vi "URL Read 3.vi"(4 "error in (no error)":errorcluster, 6 "Container State":T3, 7 "Display State In":T1={"WebView2 Ref"=refnum, "event callback refnum"=refnum, "Events"={"Navigation Complete Event"=refnum, "Source Changed Event"=refnum, "Document Title Changed Event"=refnum, "Status Bar Text Changed"=refnum, "Web Message Received"=refnum, "Window Close Requested"=refnum}, "Paths"={"Webview2 Native"=path "C:/Users/kleins/Desktop/webview2/microsoft.web.webview2.1.0.1370.28/build/native", "Edge Application"=path "", "User Data"=path ""}}) -> (0 "error out":errorcluster, 2 "Value":string, 3 "Display State Out":T1={"WebView2 Ref"=refnum, "event callback refnum"=refnum, "Events"={"Navigation Complete Event"=refnum, "Source Changed Event"=refnum, "Document Title Changed Event"=refnum, "Status Bar Text Changed"=refnum, "Web Message Received"=refnum, "Window Close Requested"=refnum}, "Paths"={"Webview2 Native"=path "C:/Users/kleins/Desktop/webview2/microsoft.web.webview2.1.0.1370.28/build/native", "Edge Application"=path "", "User Data"=path ""}})   [LabVIEW 2020, in "WebView2 Control.xctl"]
uses:
  WebView2 Control.xctl
  <vilib>/_xctls/Container State.ctl
  State.ctl
  E:/Labview/LV 2020/Libs/LV-WebView2/microsoft.web.webview2/lib/net45/Microsoft.Web.WebView2.WinForms.dll
  microsoft.web.webview2/lib/net45/Microsoft.Web.WebView2.WinForms.dll
  Paths.ctl
  <vilib>/_xctls/XControlSupport.lvlib
panel:
  # "Replace the Value Indicator below with an Indicator of desired type.\nDo not remove this Indicator or the others from the connector pane. \nDo not change the connector pane pattern.\nThe Value Indicator should always be the second terminal from top on the output side in the connector pane."
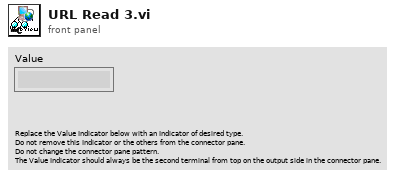
[diagram p1: front panel]
types:
  T1 = typedef "WebView2 Control.xctl/State.ctl" = cluster{"WebView2 Ref":refnum<data-value>, "event callback refnum":refnum<k27>, "Events":cluster{"Navigation Complete Event":refnum<user-event>, "Source Changed Event":refnum<user-event>, "Document Title Changed Event":refnum<user-event>, "Status Bar Text Changed":refnum<user-event>, "Web Message Received":refnum<user-event>, "Window Close Requested":refnum<user-event>}, "Paths":T2}
  T2 = typedef "WebView2 Control.xctl/Paths.ctl" = cluster{"Webview2 Native":path, "Edge Application":path, "User Data":path}
  T3 = typedef "XControlSupport.lvlib/Container State.ctl" = cluster{"Indicator?":bool, "Run Mode?":bool, " Refnum":refnum<vi>}
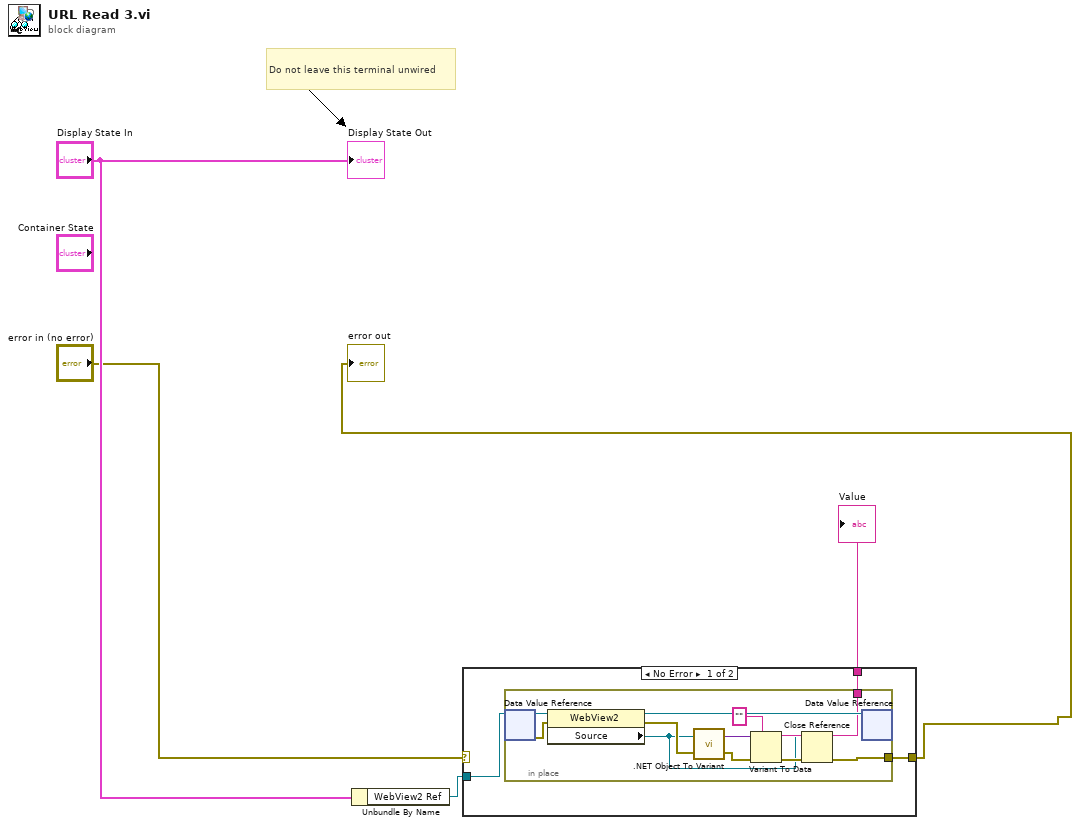
[diagram p0: block diagram]
diagram:
  # "Do not leave this terminal unwired"
  n1 = Unbundle By Name("Display State In") -> ("WebView2 Ref"=w5:refnum<data-value>)
  n2 = case shown="No Error" "error in (no error)" {
    selector: "error in (no error)" -> [_ w20]
    tunnel: [w8 w20] -> w1
    tunnel: w5 -> [w7 _]
    tunnel: [w6 _] -> w3
    frame No Error {
      n3 = in-place {
        in-place-border: [w10] -> w8
        in-place-border: [w11] -> w6
        n4 = in-place-dvr #1(w7) -> (w19:refnum<k24>, w18:errorcluster)
        n5 = property class="WebView2"(reference=w19, error in=w18) -> (reference out=w17:refnum<k24>, error out=w13:errorcluster, "Source"=w9:refnum<k24>)
        n6 = call <vilib>:".NET Object To Variant.vi"("error in (no error)"=w13, ".NET object"=w9) -> ("error out"=w16:errorcluster, "variant"=w15:variant)
        n7 = Variant To Data(error in=w16, type="", Variant=w15) -> (data=w11:string, error out=w12:errorcluster)
        n8 = Close Reference(reference=w9, error in (no error)=w12) -> (error out=w10:errorcluster)
        n9 = in-place-dvr #1(w17) -> ()  [unwired: 2 out]
      }
    }
    frame Error {
    }
  }
  "error out" <- w1
  "Value" <- w3
  "Display State Out" <- "Display State In"
